vi "Waveform to 2D Array.vi"   [LabVIEW 2016]
doc: "This function works by stepping through the array of waveform data, getting the waveform components dt (time difference between samples) and Y (amplitude of sample), then auto-indexing through the array using a for loop. Inside this loop, a 2-D array is constructed, again using auto-indexing. This new array contains time data in the first column, calculated by multiplying the dt of the waveform with the iteration of the for loop. Subsequent columns contain waveform amplitude data; there will be one additional column for each waveform in the initial array of waveforms."
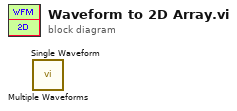
[diagram p0: block diagram]
diagram:
  n1 = call "Multiple Waveforms.vi"() -> ()  [unwired: 10 in, 2 out]
  n2 = call "Single Waveform.vi"() -> ()  [unwired: 10 in, 2 out]
